vi "minicryo_H-full_202102.vi"() -> ()   [LabVIEW 2013]
uses:
  subVI/B_Globals.vi
  <vilib>/Analysis/NI_AALPro.lvlib
panel:
  out "Numeric":i32
  out "Set Field [T]":dbl
  out "Set Rate [T]":dbl=0.21275819999999998
  out "Exec Time [ms]":u32=526
  out "Stable":bool=TRUE
  out "Act. Rate [T/min]":dbl=-2.1033442988388268e-05
  out "Read Buffer":string="45:85:76 OUTPUT: 0.00000 TESLA AT 0.0 VOLTS \r\n"
  in  "stop":bool
  out "Its":i32=853
  out "Running Sequence":bool
  in  "Set Field":dbl
  in  "Rate":dbl=0.2
  in  "Go To":bool
  out "Field [T]":dbl
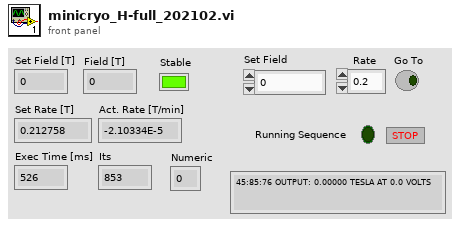
[diagram p1: front panel]
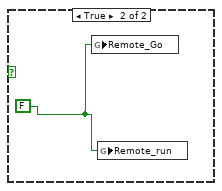
[diagram p2: hidden frame]
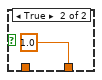
[diagram p3: hidden frame]
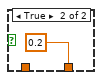
[diagram p4: hidden frame]
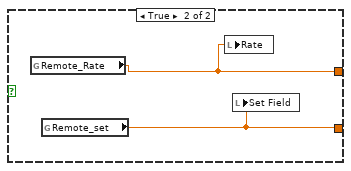
[diagram p5: hidden frame]
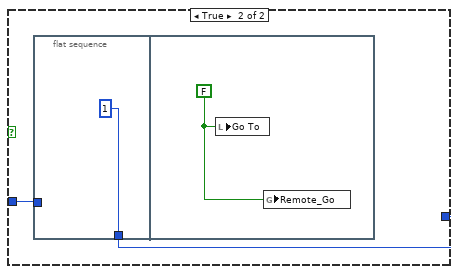
[diagram p6: hidden frame]
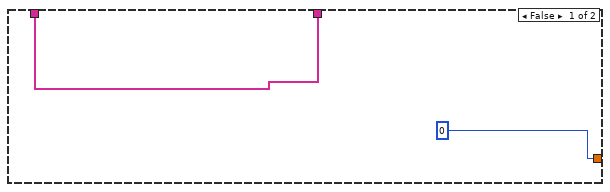
[diagram p7: hidden frame]
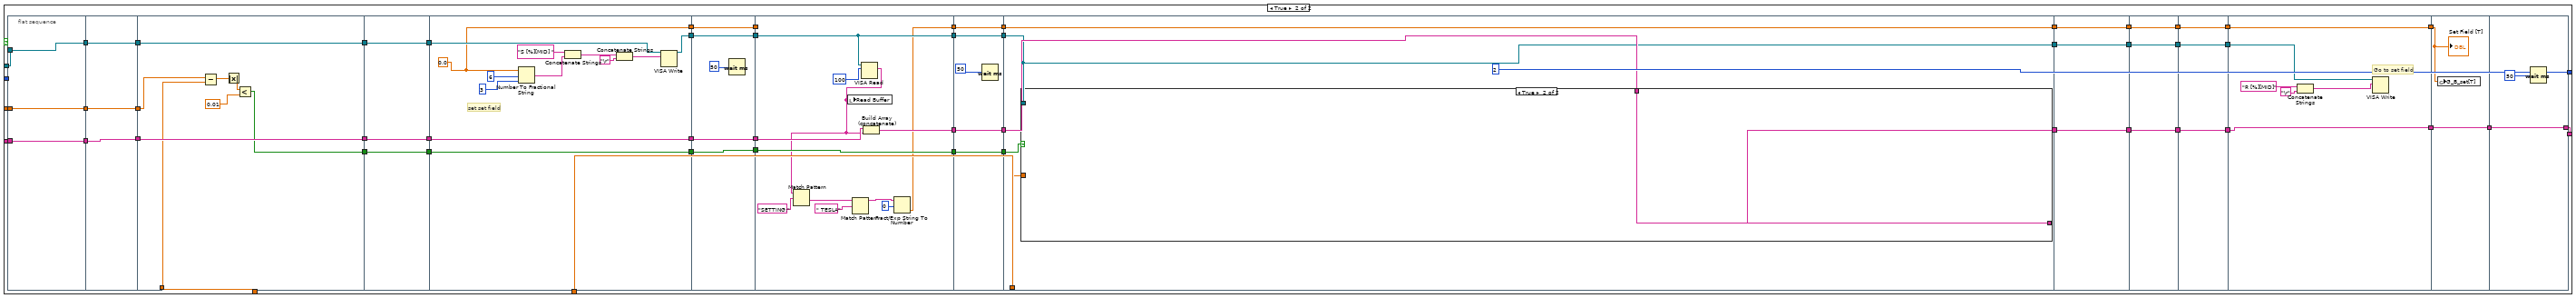
[diagram p10: hidden frame]
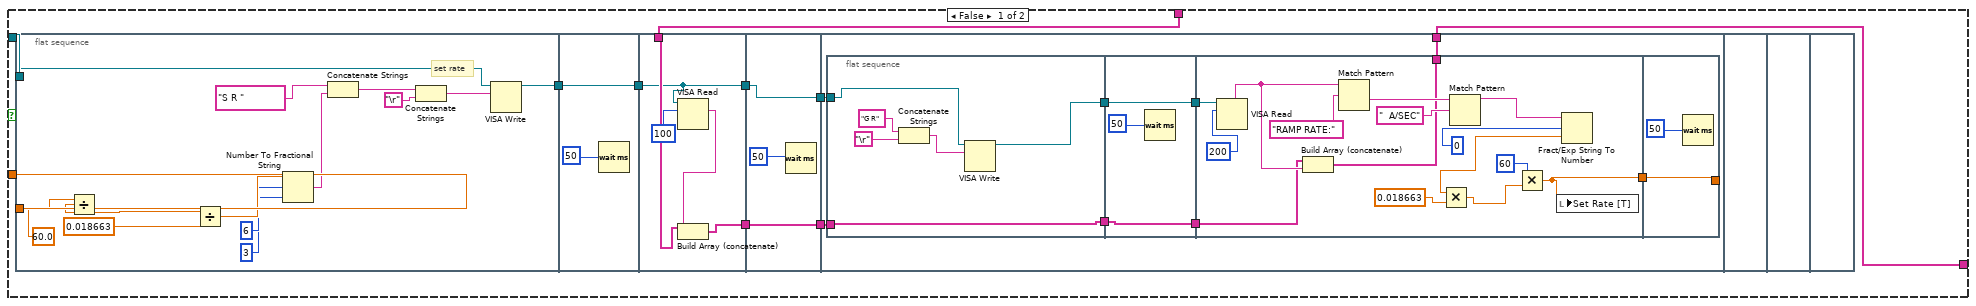
[diagram p11: hidden frame]
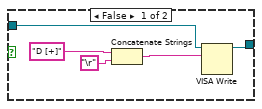
[diagram p14: hidden frame]
diagram:
  n1 = Tick Count (ms)() -> (millisecond timer value=w2:u32)
  n2 = VISA Clear(VISA resource name=refnum<visa-resource-name> "COM7" ("Lakeshore Address")) -> (VISA resource name out=w3:refnum<visa-resource-name>)  [unwired: 1 in, 1 out]
  n3 = while {
    shift-right: [w134] -> _
    shift-left: _ -> [w135]
    shift-right: [w131] -> _
    shift-left: _ -> [w132]
    tunnel: w3 -> [w136]
    shift-right: [w127] -> _
    shift-left: 0 -> [w93]
    shift-right: [w114] -> _
    shift-left: w2 -> [w113]
    shift-right: [w68] -> _
    shift-left: _ -> [w77]
    i -> [w124]
    stop <- FALSE stop-if-true
    n4 = flat-sequence {
      tunnel: w93 -> [w137]
      tunnel: w132 -> [w140]
      tunnel: w135 -> [w142]
      tunnel: w136 -> [w146]
      tunnel: [w146] -> w92
      tunnel: [w143] -> w91
      tunnel: [w139] -> w90
      tunnel: [w137] -> w89
      tunnel: [w138] -> w78
      tunnel: w77 -> [w138]
      tunnel: [w154] -> w118
      tunnel: [w153] -> w117
      tunnel: [w152] -> w116
      tunnel: [w151] -> w115
      tunnel: [w149] -> w114
      tunnel: w113 -> [w148]
      tunnel: w92 -> [w154]
      tunnel: w91 -> [w153]
      tunnel: w90 -> [w152]
      tunnel: w89 -> [w151]
      tunnel: w78 -> [w147]
      tunnel: [w147] -> w74
      tunnel: [w161] -> w88
      tunnel: [w160] -> w86
      tunnel: [w159] -> w84
      tunnel: [w158] -> w82
      tunnel: [w156] -> w80
      tunnel: w118 -> [w161]
      tunnel: w117 -> [w160]
      tunnel: w116 -> [w159]
      tunnel: w115 -> [w158]
      tunnel: [w155] -> w75
      tunnel: w74 -> [w155]
      tunnel: w88 -> [w164]
      tunnel: [w163] -> w87
      tunnel: w86 -> [w169]
      tunnel: [w169] -> w85
      tunnel: w84 -> [w168]
      tunnel: [w168] -> w83
      tunnel: w82 -> [w167]
      tunnel: [w167] -> w81
      tunnel: w80 -> [w166]
      tunnel: [w166] -> w79
      tunnel: [w165] -> w76
      tunnel: w75 -> [w165]
      tunnel: w87 -> [w170]
      tunnel: [w170] -> w123
      tunnel: w85 -> [w176]
      tunnel: [w176] -> w122
      tunnel: w83 -> [w175]
      tunnel: [w175] -> w121
      tunnel: w81 -> [w174]
      tunnel: [w174] -> w120
      tunnel: w79 -> [w173]
      tunnel: [w173] -> w119
      tunnel: w76 -> [w171]
      tunnel: [w171] -> w72
      tunnel: [w186] -> w112
      tunnel: [w185] -> w111
      tunnel: [w183] -> w110
      tunnel: [w184] -> w109
      tunnel: [w179] -> w108
      tunnel: w123 -> [w179]
      tunnel: w122 -> [w186]
      tunnel: w121 -> [w185]
      tunnel: w120 -> [w184]
      tunnel: w119 -> [w183]
      tunnel: [w178] -> w94
      tunnel: [w177] -> w73
      tunnel: w72 -> [w177]
      tunnel: w112 -> [w194]
      tunnel: [w194] -> w25
      tunnel: w111 -> [w193]
      tunnel: [w193] -> w24
      tunnel: w110 -> [w192]
      tunnel: [w192] -> w23
      tunnel: w109 -> [w191]
      tunnel: [w191] -> w22
      tunnel: w108 -> [w190]
      tunnel: [w190] -> w21
      tunnel: [w188] -> w20
      tunnel: w94 -> [w188]
      tunnel: w73 -> [w187]
      tunnel: [w187] -> w19
      tunnel: w25 -> [w201]
      tunnel: [w201] -> w18
      tunnel: w24 -> [w200]
      tunnel: [w200] -> w16
      tunnel: w23 -> [w199]
      tunnel: [w199] -> w14
      tunnel: w22 -> [w198]
      tunnel: [w198] -> w12
      tunnel: w21 -> [w197]
      tunnel: [w197] -> w10
      tunnel: w20 -> [w195]
      tunnel: [w195] -> w8
      tunnel: w19 -> [w196]
      tunnel: [w196] -> w6
      tunnel: w18 -> [w209]
      tunnel: [w209] -> w17
      tunnel: w16 -> [w208]
      tunnel: [w208] -> w15
      tunnel: w14 -> [w207]
      tunnel: [w207] -> w13
      tunnel: w12 -> [w206]
      tunnel: [w206] -> w11
      tunnel: w10 -> [w205]
      tunnel: [w205] -> w9
      tunnel: w8 -> [w204]
      tunnel: [w204] -> w7
      tunnel: w6 -> [w203]
      tunnel: [w203] -> w5
      tunnel: [w214] -> w107
      tunnel: w17 -> [w225]
      tunnel: [w225] -> w106
      tunnel: w15 -> [w224]
      tunnel: [w224] -> w105
      tunnel: w13 -> [w223]
      tunnel: [w223] -> w104
      tunnel: w11 -> [w222]
      tunnel: [w222] -> w103
      tunnel: w9 -> [w221]
      tunnel: [w221] -> w102
      tunnel: [w213] -> w101
      tunnel: w7 -> [w212]
      tunnel: [w211] -> w71
      tunnel: w5 -> [w211]
      tunnel: [w210] -> w26
      tunnel: [w235] -> w49
      tunnel: [w230] -> w48
      tunnel: [w234] -> w47
      tunnel: [w233] -> w46
      tunnel: [w232] -> w45
      tunnel: [w231] -> w44
      tunnel: w107 -> [w230]
      tunnel: w106 -> [w231]
      tunnel: w105 -> [w233]
      tunnel: w104 -> [w232]
      tunnel: w103 -> [w235]
      tunnel: w102 -> [w234]
      tunnel: w101 -> [w229]
      tunnel: w71 -> [w227]
      tunnel: [w228] -> w43
      tunnel: [w226] -> w27
      tunnel: w26 -> [w226]
      tunnel: w49 -> [w244]
      tunnel: [w244] -> w42
      tunnel: w48 -> [w243]
      tunnel: [w243] -> w40
      tunnel: w47 -> [w242]
      tunnel: [w242] -> w38
      tunnel: w46 -> [w241]
      tunnel: [w241] -> w36
      tunnel: w45 -> [w240]
      tunnel: [w240] -> w34
      tunnel: w44 -> [w239]
      tunnel: [w239] -> w32
      tunnel: w43 -> [w238]
      tunnel: [w238] -> w30
      tunnel: [w237] -> w28
      tunnel: w27 -> [w237]
      tunnel: w42 -> [w251]
      tunnel: [w251] -> w41
      tunnel: w40 -> [w250]
      tunnel: [w250] -> w39
      tunnel: w38 -> [w249]
      tunnel: [w249] -> w37
      tunnel: w36 -> [w248]
      tunnel: [w248] -> w35
      tunnel: w34 -> [w247]
      tunnel: [w247] -> w33
      tunnel: w32 -> [w246]
      tunnel: [w246] -> w31
      tunnel: w30 -> [w245]
      tunnel: [w245] -> w29
      tunnel: w28 -> [_]
      tunnel: w41 -> [w259]
      tunnel: [w259] -> w100
      tunnel: w39 -> [w258]
      tunnel: [w258] -> w99
      tunnel: w37 -> [w257]
      tunnel: [w257] -> w98
      tunnel: w35 -> [w256]
      tunnel: [w256] -> w97
      tunnel: w33 -> [w255]
      tunnel: [w255] -> w96
      tunnel: w31 -> [w254]
      tunnel: [w254] -> w95
      tunnel: [w252] -> w70
      tunnel: w29 -> [w252]
      tunnel: [w280] -> w130
      tunnel: [w278] -> w129
      tunnel: [w288] -> w128
      tunnel: w100 -> [w288]
      tunnel: [w283] -> w126
      tunnel: w99 -> [w283]
      tunnel: [w287] -> w125
      tunnel: w98 -> [w287]
      tunnel: w97 -> [w286]
      tunnel: w96 -> [w285]
      tunnel: w95 -> [w284]
      tunnel: w70 -> [w270]
      tunnel: [w270] -> w69
      tunnel: w130 -> [w307]
      tunnel: w129 -> [w306]
      tunnel: w128 -> [w302]
      tunnel: [w307] -> w67
      tunnel: [w306] -> w65
      tunnel: [w301] -> w63
      tunnel: [w300] -> w61
      tunnel: w126 -> [w300]
      tunnel: w125 -> [w299]
      tunnel: [w299] -> w59
      tunnel: [w289] -> w57
      tunnel: [w293] -> w55
      tunnel: [w297] -> w53
      tunnel: w69 -> [w297]
      tunnel: w67 -> [w335]
      tunnel: [w335] -> w66
      tunnel: w65 -> [w334]
      tunnel: [w334] -> w64
      tunnel: w63 -> [w324]
      tunnel: [w324] -> w62
      tunnel: w61 -> [w333]
      tunnel: [w333] -> w60
      tunnel: w59 -> [w330]
      tunnel: [w330] -> w58
      tunnel: w57 -> [w332]
      tunnel: [w332] -> w56
      tunnel: w55 -> [w331]
      tunnel: [w331] -> w54
      tunnel: w53 -> [w329]
      tunnel: [w328] -> w52
      tunnel: [w326] -> w51
      tunnel: [w321] -> w50
      tunnel: [w379] -> w131
      tunnel: [w380] -> w134
      tunnel: w66 -> [w380]
      tunnel: w64 -> [w379]
      tunnel: w62 -> [w373]
      tunnel: [w378] -> w127
      tunnel: w60 -> [w377]
      tunnel: w58 -> [w376]
      tunnel: w56 -> [w375]
      tunnel: w54 -> [w374]
      tunnel: [w372] -> w68
      tunnel: w52 -> [w371]
      tunnel: w51 -> [w370]
      tunnel: w50 -> [w369]
      frame #0 {
        n5 = Array Size(array=w142) -> (size(s)=w145:i32)
        n6 = Subtract(x=w145, y=1000) -> (x-y=w141:i32)
        n7 = Array Subset(array=w142, index=w141) -> (w143:dbl[])  [unwired: 1 in]
        n8 = Array Subset(array=w140, index=w141) -> (w139:dbl[])  [unwired: 1 in]
        "Numeric" <- w137
      }
      frame #1 {
        n9 = Tick Count (ms)() -> (millisecond timer value=w149:u32)
        n10 = Subtract(x=w149, y=w148) -> (x-y=→"Exec Time [ms]":u32)
      }
      frame #2 {
        n11 = case shown="False" "stop" {
          frame False {
          }
          frame True {
            w162 = FALSE
            n12 = global write "B_Globals.vi" "Remote_Go"(w162) -> ()
            n13 = global write "B_Globals.vi" "Remote_run"(w162) -> ()
          }
        }
        n14 = call <vilib>:"High Resolution Relative Seconds.vi"() -> ("relative seconds"=w156:dbl)
      }
      frame #3 {
        n15 = VISA Clear(VISA resource name=w164) -> (VISA resource name out=w163:refnum<visa-resource-name>)  [unwired: 1 in, 1 out]
      }
      frame #4 {
        n16 = Wait (ms)(milliseconds to wait=u32 20 ("Pre Delay")) -> ()  [unwired: 1 out]
      }
      frame #5 {
        n17 = Concatenate Strings("GET OUTPUT " ("Command"), "\r") -> (w181:string)
        n18 = VISA Write(VISA resource name=w179, write buffer=w181) -> (VISA resource name out=w178:refnum<visa-resource-name>)  [unwired: 1 in, 2 out]
      }
      frame #6 {
        n19 = Wait (ms)(milliseconds to wait=u32 50 ("Pre Delay")) -> ()  [unwired: 1 out]
      }
      frame #7 {
      }
      frame #8 {
        n20 = Wait (ms)(milliseconds to wait=u32 50 ("Pre Delay")) -> ()  [unwired: 1 out]
      }
      frame #9 {
        n21 = VISA Read(VISA resource name=w212, byte count=u32 100) -> (VISA resource name out=w210:refnum<visa-resource-name>, read buffer=w213:string)  [unwired: 1 in, 2 out]
        n22 = Match Pattern(string=w213, regular expression="OUTPUT:") -> (after substring=w216:string)  [unwired: 1 in, 3 out]
        n23 = Match Pattern(string=w216, regular expression=" TESLA") -> (before substring=w215:string)  [unwired: 1 in, 3 out]
        n24 = Fract/Exp String To Number(string=w215, offset=0) -> (number=w214:dbl)  [unwired: 2 in, 1 out]
      }
      frame #10 {
        n25 = global write "B_Globals.vi" "B [T]"(w230) -> ()
        n26 = Build Array (concatenate)(w227, w229) -> (w228:string[])
        "Field [T]" <- w230
        "Read Buffer" <- w229
      }
      frame #11 {
        n27 = Wait (ms)(milliseconds to wait=u32 0 ("Pre Delay")) -> ()  [unwired: 1 out]
      }
      frame #12 {
      }
      frame #13 {
        n28 = Wait (ms)(milliseconds to wait=u32 100 ("Pre Delay")) -> ()  [unwired: 1 out]
      }
      frame #14 {
        n29 = Build Array (concatenate)(w284, w283) -> (w280:dbl[])
        n30 = Build Array (concatenate)(w286, w285) -> (w278:dbl[])
        n31 = Array Size(array=w280) -> (size(s)=w281:i32)
        n32 = Subtract(x=w281, y=50) -> (x-y=w279:i32)
        n33 = Array Subset(array=w278, index=w279) -> (w276:dbl[])  [unwired: 1 in]
        n34 = Array Subset(array=w280, index=w279) -> (w277:dbl[])  [unwired: 1 in]
        n35 = call <vilib>:"Linear Fit.vi"("Y"=w277, "X"=w276) -> ("slope"=w272:dbl)  [unwired: 9 in, 4 out]
        n36 = local read "Set Field [T]"() -> (w263:dbl)
        n37 = local read "Field [T]"() -> (w262:dbl)
        n38 = Multiply(x=w272, y=60) -> (x*y=w271:dbl)
        "Act. Rate [T/min]" <- w271
        n39 = Absolute Value(x=w263) -> (abs(x)=w260:dbl)
        n40 = Absolute Value(x=w262) -> (abs(x)=w261:dbl)
        n41 = Subtract(x=w260, y=w261) -> (x-y=w269:dbl)
        n42 = Absolute Value(x=w271) -> (abs(x)=w273:dbl)
        n43 = Less?(x=w273, y=0.01) -> (x < y?=w265:bool)
        n44 = Absolute Value(x=w269) -> (abs(x)=w268:dbl)
        n45 = Less?(x=w268, y=0.02) -> (x < y?=w264:bool)
        n46 = And(x=w265, y=w264) -> (x .and. y?=w266:bool)
        "Stable" <- w266
        n47 = global write "B_Globals.vi" "Rem_stable_B"(w266) -> ()
      }
      frame #15 {
        n48 = global read "B_Globals.vi" "Remote_Go"() -> (w305:bool)
        n49 = global read "B_Globals.vi" "Remote_run"() -> (w298:bool)
        "Running Sequence" <- w298
        n50 = Or(x=w305, y="Go To") -> (x .or. y?=w303:bool)
        n51 = case shown="False" w303 {
          tunnel: w302 -> [w316 w318]
          tunnel: [w316 w317] -> w301
          frame False {
          }
          frame True {
            n52 = flat-sequence {
              tunnel: w318 -> [_]
              tunnel: [1] -> w317
              frame #0 {
              }
              frame #1 {
                w320 = FALSE
                n53 = local write "Go To"(w320) -> ()
                n54 = global write "B_Globals.vi" "Remote_Go"(w320) -> ()
              }
            }
          }
        }
        n55 = case shown="False" w298 {
          tunnel: ["Set Field" w314] -> w290
          tunnel: ["Rate" w315] -> w294
          frame False {
          }
          frame True {
            n56 = global read "B_Globals.vi" "Remote_Rate"() -> (w315:dbl)
            n57 = global read "B_Globals.vi" "Remote_set"() -> (w314:dbl)
            n58 = local write "Rate"(w315) -> ()
            n59 = local write "Set Field"(w314) -> ()
          }
        }
        n60 = Greater?(x=w294, y=0.2) -> (0:w295:bool)
        n61 = Greater?(x=w290, y=1.0) -> (0:w291:bool)
        n62 = case shown="False" w291 {
          tunnel: [w308 1.0] -> w289
          tunnel: w290 -> [w308 _]
          frame False {
          }
          frame True {
          }
        }
        n63 = case shown="False" w295 {
          tunnel: [w310 0.2] -> w293
          tunnel: w294 -> [w310 _]
          frame False {
          }
          frame True {
          }
        }
      }
      frame #16 {
        n64 = Not Equal?(x=0, y=w324) -> (x != y?=w321:bool)
        n65 = Not Equal?(x=w324, y=2) -> (x != y?=w323:bool)
        n66 = And(x=w323, y=w321) -> (x .and. y?=w322:bool)
        n67 = case shown="True" w322 {
          tunnel: w330 -> [_ w342]
          tunnel: w329 -> [w337 w341]
          tunnel: [w337 w340] -> w328
          tunnel: [0 w338] -> w326
          frame False {
          }
          frame True {
            n68 = flat-sequence {
              tunnel: w342 -> [w346]
              tunnel: [w345] -> w344
              tunnel: w344 -> [w350]
              tunnel: [w350] -> w343
              tunnel: w343 -> [w363]
              tunnel: w341 -> [w360]
              tunnel: [w359] -> w340
              tunnel: [w352] -> w339
              tunnel: [w367] -> w338
              tunnel: w339 -> [w367]
              frame #0 {
                n69 = Concatenate Strings("G R" ("Command"), "\r") -> (w348:string)
                n70 = VISA Write(VISA resource name=w346, write buffer=w348) -> (VISA resource name out=w345:refnum<visa-resource-name>)  [unwired: 1 in, 2 out]
              }
              frame #1 {
                n71 = Wait (ms)(milliseconds to wait=100) -> ()  [unwired: 1 out]
              }
              frame #2 {
                (unwired) 0.018663 ("y")
                n72 = VISA Read(VISA resource name=w363, byte count=u32 200) -> (read buffer=w361:string)  [unwired: 1 in, 3 out]
                n73 = Build Array (concatenate)(w360, w361) -> (w359:string[])
                n74 = Match Pattern(string=w361, regular expression="RAMP RATE:") -> (after substring=w364:string)  [unwired: 1 in, 3 out]
                n75 = Match Pattern(string=w364, regular expression="  A/SEC") -> (before substring=w357:string)  [unwired: 1 in, 3 out]
                n76 = Fract/Exp String To Number(string=w357, offset=0) -> (number=w355:dbl)  [unwired: 2 in, 1 out]
                n77 = Multiply(x=w355, y=0.018663) -> (x*y=w353:dbl)
                n78 = Multiply(x=60, y=w353) -> (x*y=w352:dbl)
                "Set Rate [T]" <- w352
              }
              frame #3 {
                n79 = Wait (ms)(milliseconds to wait=100) -> ()  [unwired: 1 out]
              }
            }
          }
        }
      }
      frame #17 {
        # "Bnow"
        # "Barray"
        n80 = case shown="3" w373 {
          tunnel: w377 -> [_ w399 w606 _ _]
          tunnel: w373 -> [w383 w392 w603 _ _]
          tunnel: [w383 w391 w602 4 w715] -> w378
          tunnel: w374 -> [_ w384 _ _ w717]
          tunnel: w376 -> [_ w388 _ w625 w713]
          tunnel: w375 -> [_ w389 _ _ w714]
          tunnel: w371 -> [w381 w387 w601 w621 w698]
          tunnel: [w381 w386 w601 w626 w692] -> w372
          tunnel: w370 -> [_ w385 _ _ _]
          tunnel: w369 -> [_ _ _ _ _]
          frame 0, Default {
            n81 = Wait (ms)(milliseconds to wait=0) -> ()  [unwired: 1 out]
          }
          frame 1 {
            # "If True need to reverse polarity"
            n82 = Less Than 0?(x=w389) -> (x < 0?=w390:bool)
            n83 = Number To Fractional String(number=w399) -> (F-format string=w402:string)  [unwired: 3 in]
            n84 = String Subset(string=w402, length (rest)=1 ("length (rest)")) -> (substring=w401:string)  [unwired: 1 in]
            n85 = Equal?(x=w401, y="-") -> (x = y?=w394:bool)
            n86 = Not Or(1:w390, 2:w394) -> (0:w398:bool)
            n87 = Not Or(1:w398, 2:w394) -> (0:w397:bool)
            n88 = Not Or(1:w390, 2:w398) -> (0:w396:bool)
            n89 = Not Or(1:w396, 2:w397) -> (0:w395:bool)
            n90 = Not(x=w395) -> (.not. x?=w393:bool)
            n91 = case shown="False" w393 {
              tunnel: w392 -> [_ _]
              tunnel: [4 2] -> w391
              tunnel: w384 -> [_ w453]
              tunnel: w388 -> [_ w451]
              tunnel: w387 -> [w404 w442]
              tunnel: [w404 w433] -> w386
              tunnel: w385 -> [_ w414]
              tunnel: w384 -> [_ w412]
              frame False {
              }
              frame True {
                n92 = flat-sequence {
                  tunnel: w451 -> [w457]
                  tunnel: [w457] -> w450
                  tunnel: [w458] -> w443
                  tunnel: w442 -> [w458]
                  tunnel: [w456] -> w415
                  tunnel: w414 -> [w456]
                  tunnel: [w461] -> w421
                  tunnel: w450 -> [w461]
                  tunnel: w443 -> [w460]
                  tunnel: [w460] -> w420
                  tunnel: w415 -> [w459]
                  tunnel: [w459] -> w413
                  tunnel: w421 -> [w469]
                  tunnel: [w469] -> w419
                  tunnel: w420 -> [w468]
                  tunnel: [w468] -> w417
                  tunnel: w413 -> [w467]
                  tunnel: w412 -> [w466]
                  tunnel: [w462] -> w411
                  tunnel: w419 -> [w472]
                  tunnel: [w472] -> w418
                  tunnel: w417 -> [w471]
                  tunnel: [w471] -> w416
                  tunnel: w411 -> [w470]
                  tunnel: [w470] -> w410
                  tunnel: [w477] -> w454
                  tunnel: w418 -> [w476]
                  tunnel: [w475] -> w440
                  tunnel: w416 -> [w475]
                  tunnel: [w474] -> w422
                  tunnel: w410 -> [w473]
                  tunnel: [w473] -> w409
                  tunnel: [w488] -> w449
                  tunnel: w454 -> [w488]
                  tunnel: [w487] -> w441
                  tunnel: w440 -> [w487]
                  tunnel: [w486] -> w423
                  tunnel: w422 -> [w486]
                  tunnel: w409 -> [w485]
                  tunnel: [w485] -> w408
                  tunnel: w449 -> [w500]
                  tunnel: [w500] -> w448
                  tunnel: w441 -> [w499]
                  tunnel: [w498] -> w438
                  tunnel: [w490] -> w424
                  tunnel: w423 -> [_]
                  tunnel: w408 -> [w497]
                  tunnel: [w497] -> w407
                  tunnel: w448 -> [w506]
                  tunnel: [w506] -> w447
                  tunnel: [w504] -> w439
                  tunnel: w438 -> [w504]
                  tunnel: [w503] -> w425
                  tunnel: w424 -> [w503]
                  tunnel: w407 -> [w502]
                  tunnel: [w502] -> w406
                  tunnel: w447 -> [w507]
                  tunnel: w453 -> [w512]
                  tunnel: [w507] -> w452
                  tunnel: w439 -> [w508]
                  tunnel: [w509] -> w436
                  tunnel: [w511] -> w426
                  tunnel: w425 -> [w511]
                  tunnel: w406 -> [w510]
                  tunnel: [w584] -> w446
                  tunnel: w452 -> [w584]
                  tunnel: [w583] -> w437
                  tunnel: w436 -> [w583]
                  tunnel: [w582] -> w427
                  tunnel: w426 -> [w582]
                  tunnel: w446 -> [w587]
                  tunnel: [w587] -> w445
                  tunnel: w437 -> [w585]
                  tunnel: [w585] -> w434
                  tunnel: [w586] -> w428
                  tunnel: w427 -> [w586]
                  tunnel: w445 -> [w590]
                  tunnel: [w590] -> w444
                  tunnel: [w589] -> w435
                  tunnel: w434 -> [w589]
                  tunnel: [w588] -> w429
                  tunnel: w428 -> [w588]
                  tunnel: w444 -> [w593]
                  tunnel: w435 -> [w592]
                  tunnel: [w592] -> w432
                  tunnel: [w591] -> w430
                  tunnel: w429 -> [w591]
                  tunnel: w432 -> [w598]
                  tunnel: [w598] -> w431
                  tunnel: w430 -> [w597]
                  tunnel: [w599] -> w433
                  tunnel: w431 -> [w599]
                  frame #0 {
                  }
                  frame #1 {
                  }
                  frame #2 {
                    n93 = Subtract(x=w467, y=w466) -> (x-y=w465:dbl)
                    n94 = Absolute Value(x=w465) -> (abs(x)=w464:dbl)
                    n95 = Less?(x=w464, y=0.01) -> (x < y?=w462:bool)
                  }
                  frame #3 {
                  }
                  frame #4 {
                    w474 = 0.0
                    # "set set field"
                    n96 = Number To Fractional String(number=w474, width (-)=i16 6, precision (6)=i16 3) -> (F-format string=w481:string)  [unwired: 1 in]
                    n97 = Concatenate Strings("S [%][MID] " ("string"), w481) -> (w478:string)
                    n98 = Concatenate Strings(w478, "\r") -> (w480:string)
                    n99 = VISA Write(VISA resource name=w476, write buffer=w480) -> (VISA resource name out=w477:refnum<visa-resource-name>)  [unwired: 1 in, 2 out]
                  }
                  frame #5 {
                    n100 = Wait (ms)(milliseconds to wait=50) -> ()  [unwired: 1 out]
                  }
                  frame #6 {
                    n101 = VISA Read(VISA resource name=w500, byte count=100) -> (read buffer=w491:string)  [unwired: 1 in, 3 out]
                    n102 = Match Pattern(string=w491, regular expression="SETTING:") -> (after substring=w495:string)  [unwired: 1 in, 3 out]
                    n103 = local write "Read Buffer"(w491) -> ()
                    n104 = Match Pattern(string=w495, regular expression=" TESLA") -> (before substring=w496:string)  [unwired: 1 in, 3 out]
                    n105 = Build Array (concatenate)(w499, w491) -> (w498:string[])
                    n106 = Fract/Exp String To Number(string=w496, offset=0) -> (number=w490:dbl)  [unwired: 2 in, 1 out]
                  }
                  frame #7 {
                    n107 = Wait (ms)(milliseconds to wait=50) -> ()  [unwired: 1 out]
                  }
                  frame #8 {
                    n108 = case shown="True" w510 {
                      tunnel: w507 -> [w522 _]
                      tunnel: w512 -> [w521 _]
                      tunnel: w508 -> [w517 w581]
                      tunnel: [w514 w581] -> w509
                      frame False {
                        n109 = flat-sequence {
                          tunnel: w522 -> [w525]
                          tunnel: w521 -> [w524]
                          tunnel: [w523] -> w520
                          tunnel: w520 -> [w538]
                          tunnel: [w538] -> w519
                          tunnel: w519 -> [w540]
                          tunnel: [w540] -> w518
                          tunnel: w517 -> [w541]
                          tunnel: [w539] -> w515
                          tunnel: w518 -> [w544]
                          tunnel: [w545] -> w516
                          tunnel: w515 -> [w545]
                          tunnel: [w544] -> w513
                          tunnel: w516 -> [w551]
                          tunnel: [w548] -> w514
                          tunnel: w513 -> [w547]
                          frame #0 {
                            # "set rate"
                            n110 = Divide(x=w524, y=60.0) -> (x/y=w530:dbl)
                            n111 = Divide(x=w530, y=0.018663) -> (x/y=w528:dbl)
                            n112 = Number To Fractional String(number=w528, width (-)=i16 6, precision (6)=i16 3) -> (F-format string=w533:string)  [unwired: 1 in]
                            n113 = Concatenate Strings("S R " ("string"), w533) -> (w532:string)
                            n114 = Concatenate Strings(w532, "\r") -> (w536:string)
                            n115 = VISA Write(VISA resource name=w525, write buffer=w536) -> (VISA resource name out=w523:refnum<visa-resource-name>)  [unwired: 1 in, 2 out]
                          }
                          frame #1 {
                            n116 = Wait (ms)(milliseconds to wait=50) -> ()  [unwired: 1 out]
                          }
                          frame #2 {
                            n117 = VISA Read(VISA resource name=w540, byte count=100) -> (read buffer=w542:string)  [unwired: 1 in, 3 out]
                            n118 = Build Array (concatenate)(w541, w542) -> (w539:string[])
                          }
                          frame #3 {
                            n119 = Wait (ms)(milliseconds to wait=50) -> ()  [unwired: 1 out]
                          }
                          frame #4 {
                            n120 = flat-sequence {
                              tunnel: [w557] -> w554
                              tunnel: w551 -> [w556]
                              tunnel: [w556] -> w549
                              tunnel: w547 -> [w555]
                              tunnel: w554 -> [w562]
                              tunnel: [w562] -> w553
                              tunnel: [w561] -> w550
                              tunnel: w549 -> [w561]
                              tunnel: w553 -> [w575]
                              tunnel: [w572] -> w548
                              tunnel: [w565] -> w552
                              tunnel: w550 -> [w564]
                              tunnel: [w579] -> _
                              tunnel: w552 -> [w579]
                              frame #0 {
                                n121 = Concatenate Strings("G R" ("Command"), "\r") -> (w559:string)
                                n122 = VISA Write(VISA resource name=w555, write buffer=w559) -> (VISA resource name out=w557:refnum<visa-resource-name>)  [unwired: 1 in, 2 out]
                              }
                              frame #1 {
                                n123 = Wait (ms)(milliseconds to wait=50) -> ()  [unwired: 1 out]
                              }
                              frame #2 {
                                n124 = VISA Read(VISA resource name=w575, byte count=u32 200) -> (read buffer=w573:string)  [unwired: 1 in, 3 out]
                                n125 = Build Array (concatenate)(w564, w573) -> (w572:string[])
                                n126 = Match Pattern(string=w573, regular expression="RAMP RATE:") -> (after substring=w576:string)  [unwired: 1 in, 3 out]
                                n127 = Match Pattern(string=w576, regular expression="  A/SEC") -> (before substring=w570:string)  [unwired: 1 in, 3 out]
                                n128 = Fract/Exp String To Number(string=w570, offset=0) -> (number=w568:dbl)  [unwired: 2 in, 1 out]
                                n129 = Multiply(x=w568, y=0.018663) -> (x*y=w566:dbl)
                                n130 = Multiply(x=60, y=w566) -> (x*y=w565:dbl)
                                n131 = local write "Set Rate [T]"(w565) -> ()
                              }
                              frame #3 {
                                n132 = Wait (ms)(milliseconds to wait=50) -> ()  [unwired: 1 out]
                              }
                            }
                          }
                          frame #5 {
                          }
                          frame #6 {
                          }
                          frame #7 {
                          }
                        }
                      }
                      frame True {
                      }
                    }
                  }
                  frame #9 {
                  }
                  frame #10 {
                  }
                  frame #11 {
                  }
                  frame #12 {
                    # "Go to set field"
                    n133 = Concatenate Strings("R [%][MID]" ("data"), "\r") -> (w596:string)
                    n134 = VISA Write(VISA resource name=w593, write buffer=w596) -> ()  [unwired: 1 in, 3 out]
                  }
                  frame #13 {
                    n135 = global write "B_Globals.vi" "G_B_set[T]"(w597) -> ()
                    "Set Field [T]" <- w597
                  }
                  frame #14 {
                    n136 = Wait (ms)(milliseconds to wait=50) -> ()  [unwired: 1 out]
                  }
                }
              }
            }
          }
          frame 2 {
            # "Awaiting 0 Field"
            n137 = Subtract(x=w606, y=0) -> (x-y=w608:dbl)
            n138 = Absolute Value(x=w608) -> (abs(x)=w605:dbl)
            n139 = Less?(x=w605, y=0.001) -> (x < y?=w604:bool)
            n140 = case shown="True" w604 {
              tunnel: w603 -> [w610 _]
              tunnel: [w610 3] -> w602
              frame False {
              }
              frame True {
                # "Close to 0"
                n141 = Wait (ms)(milliseconds to wait=1000) -> ()  [unwired: 1 out]
              }
            }
          }
          frame 3 {
            n142 = flat-sequence {
              tunnel: w625 -> [w630]
              tunnel: [w630] -> w624
              tunnel: w624 -> [w636]
              tunnel: [w635] -> w623
              tunnel: w623 -> [w638]
              tunnel: [w638] -> w622
              tunnel: w622 -> [w648]
              tunnel: [w648] -> w618
              tunnel: w621 -> [w646]
              tunnel: [w645] -> w616
              tunnel: [w641] -> w613
              tunnel: w618 -> [w652]
              tunnel: [w652] -> w617
              tunnel: w616 -> [w651]
              tunnel: [w651] -> w615
              tunnel: [w649] -> w614
              tunnel: w613 -> [w649]
              tunnel: [w657] -> w628
              tunnel: w617 -> [w658]
              tunnel: w615 -> [w656]
              tunnel: [w656] -> w620
              tunnel: w614 -> [w654]
              tunnel: w628 -> [w671]
              tunnel: [w671] -> w627
              tunnel: w620 -> [w669]
              tunnel: [w669] -> w619
              tunnel: w627 -> [w676]
              tunnel: [w674] -> w626
              tunnel: w619 -> [w672]
              frame #0 {
                n143 = Wait (ms)(milliseconds to wait=500) -> ()  [unwired: 1 out]
              }
              frame #1 {
                n144 = Concatenate Strings("GET S " ("data"), "\r") -> (w632:string)
                n145 = VISA Write(VISA resource name=w636, write buffer=w632) -> (VISA resource name out=w635:refnum<visa-resource-name>)  [unwired: 1 in, 2 out]
              }
              frame #2 {
                n146 = Wait (ms)(milliseconds to wait=50) -> ()  [unwired: 1 out]
              }
              frame #3 {
                n147 = VISA Read(VISA resource name=w648, byte count=100) -> (read buffer=w644:string)  [unwired: 1 in, 3 out]
                n148 = local write "Read Buffer"(w644) -> ()
                n149 = Build Array (concatenate)(w646, w644) -> (w645:string[])
                n150 = Match Pattern(string=w644, regular expression="CURRENT DIRECTION: ") -> (after substring=w642:string)  [unwired: 1 in, 3 out]
                n151 = Search and Replace String(input string=w642, search string="\r\n", replace string="") -> (result string=w641:string)  [unwired: 5 in, 3 out]
              }
              frame #4 {
                n152 = Wait (ms)(milliseconds to wait=50) -> ()  [unwired: 1 out]
              }
              frame #5 {
                (unwired) TRUE
                # "Switch polarity"
                n153 = Equal?(x=w654, y="POSITIVE") -> (x = y?=w653:bool)
                n154 = case shown="True" w653 {
                  tunnel: w658 -> [w659 w665]
                  tunnel: [w660 w664] -> w657
                  frame False {
                    n155 = Concatenate Strings("D [+]" ("data"), "\r") -> (w663:string)
                    n156 = VISA Write(VISA resource name=w659, write buffer=w663) -> (VISA resource name out=w660:refnum<visa-resource-name>)  [unwired: 1 in, 2 out]
                  }
                  frame True {
                    n157 = Concatenate Strings("D [-]" ("data"), "\r") -> (w668:string)
                    n158 = VISA Write(VISA resource name=w665, write buffer=w668) -> (VISA resource name out=w664:refnum<visa-resource-name>)  [unwired: 1 in, 2 out]
                  }
                }
              }
              frame #6 {
                n159 = Wait (ms)(milliseconds to wait=50) -> ()  [unwired: 1 out]
              }
              frame #7 {
                n160 = VISA Read(VISA resource name=w676, byte count=100) -> (read buffer=w673:string)  [unwired: 1 in, 3 out]
                n161 = Build Array (concatenate)(w672, w673) -> (w674:string[])
                n162 = local write "Read Buffer"(w673) -> ()
              }
              frame #8 {
                n163 = Wait (ms)(milliseconds to wait=500) -> ()  [unwired: 1 out]
              }
            }
          }
          frame 4 {
            n164 = flat-sequence {
              tunnel: w713 -> [w720]
              tunnel: [w720] -> w711
              tunnel: [w719] -> w700
              tunnel: w698 -> [w719]
              tunnel: [w722] -> w712
              tunnel: w711 -> [w722]
              tunnel: w700 -> [w721]
              tunnel: [w721] -> w699
              tunnel: [w726] -> w718
              tunnel: w714 -> [w724]
              tunnel: w712 -> [w727]
              tunnel: [w725] -> w702
              tunnel: w699 -> [w725]
              tunnel: [w724] -> w686
              tunnel: [w737] -> w710
              tunnel: w718 -> [w737]
              tunnel: w702 -> [w736]
              tunnel: [w736] -> w701
              tunnel: [w735] -> w687
              tunnel: w686 -> [w735]
              tunnel: w710 -> [w749]
              tunnel: [w749] -> w709
              tunnel: [w747] -> w704
              tunnel: w701 -> [w746]
              tunnel: w687 -> [_]
              tunnel: [w739] -> w678
              tunnel: [w754] -> w682
              tunnel: [w753] -> w681
              tunnel: [w752] -> w680
              tunnel: [w751] -> w679
              tunnel: w717 -> [w751]
              tunnel: w704 -> [w753]
              tunnel: w709 -> [w754]
              tunnel: w678 -> [w752]
              tunnel: w682 -> [w763]
              tunnel: [w763] -> w685
              tunnel: w681 -> [w762]
              tunnel: [w761] -> w684
              tunnel: w680 -> [w764]
              tunnel: [w764] -> w683
              tunnel: w679 -> [w756]
              tunnel: w685 -> [w834]
              tunnel: [w834] -> w706
              tunnel: [w833] -> w703
              tunnel: w684 -> [w833]
              tunnel: [w832] -> w688
              tunnel: w683 -> [w832]
              tunnel: w706 -> [w837]
              tunnel: [w837] -> w705
              tunnel: w703 -> [w836]
              tunnel: [w836] -> w693
              tunnel: [w835] -> w689
              tunnel: w688 -> [w835]
              tunnel: [w840] -> w716
              tunnel: w705 -> [w840]
              tunnel: [w839] -> w694
              tunnel: w693 -> [w839]
              tunnel: [w838] -> w690
              tunnel: w689 -> [w838]
              tunnel: w716 -> [w845]
              tunnel: [0] -> w715
              tunnel: [w843] -> w707
              tunnel: [w842] -> w695
              tunnel: w694 -> [w842]
              tunnel: [w841] -> w691
              tunnel: w690 -> [w841]
              tunnel: [w851] -> w708
              tunnel: w707 -> [w851]
              tunnel: [w850] -> w696
              tunnel: w695 -> [w850]
              tunnel: w691 -> [w849]
              tunnel: w708 -> [_]
              tunnel: [w853] -> w697
              tunnel: w696 -> [w853]
              tunnel: [w854] -> w692
              tunnel: w697 -> [w854]
              frame #0 {
              }
              frame #1 {
                n165 = Wait (ms)(milliseconds to wait=50) -> ()  [unwired: 1 out]
              }
              frame #2 {
                # "set set field"
                n166 = Number To Fractional String(number=w724, width (-)=i16 6, precision (6)=i16 3) -> (F-format string=w731:string)  [unwired: 1 in]
                n167 = Concatenate Strings("S [%][MID] " ("string"), w731) -> (w728:string)
                n168 = Concatenate Strings(w728, "\r") -> (w730:string)
                n169 = VISA Write(VISA resource name=w727, write buffer=w730) -> (VISA resource name out=w726:refnum<visa-resource-name>)  [unwired: 1 in, 2 out]
              }
              frame #3 {
                n170 = Wait (ms)(milliseconds to wait=50) -> ()  [unwired: 1 out]
              }
              frame #4 {
                n171 = VISA Read(VISA resource name=w749, byte count=100) -> (read buffer=w740:string)  [unwired: 1 in, 3 out]
                n172 = Build Array (concatenate)(w746, w740) -> (w747:string[])
                n173 = local write "Read Buffer"(w740) -> ()
                n174 = Match Pattern(string=w740, regular expression="SETTING:") -> (after substring=w744:string)  [unwired: 1 in, 3 out]
                n175 = Match Pattern(string=w744, regular expression=" TESLA") -> (before substring=w745:string)  [unwired: 1 in, 3 out]
                n176 = Fract/Exp String To Number(string=w745, offset=0) -> (number=w739:dbl)  [unwired: 2 in, 1 out]
              }
              frame #5 {
                n177 = Wait (ms)(milliseconds to wait=50) -> ()  [unwired: 1 out]
              }
              frame #6 {
                n178 = local read "Set Rate [T]"() -> (w757:dbl)
                n179 = Subtract(x=w757, y=w756) -> (x-y=w760:dbl)
                n180 = Absolute Value(x=w760) -> (abs(x)=w759:dbl)
                n181 = Less?(x=w759, y=0.01) -> (x < y?=w755:bool)
                n182 = case shown="False" w755 {
                  tunnel: w763 -> [w774 _]
                  tunnel: w756 -> [w773 _]
                  tunnel: [w767 w831] -> w761
                  tunnel: w762 -> [w765 w831]
                  frame False {
                    n183 = flat-sequence {
                      tunnel: w774 -> [w777]
                      tunnel: w773 -> [w776]
                      tunnel: [w775] -> w772
                      tunnel: w772 -> [w790]
                      tunnel: [w790] -> w771
                      tunnel: w771 -> [w793]
                      tunnel: [w793] -> w770
                      tunnel: [w792] -> w768
                      tunnel: w765 -> [w791]
                      tunnel: w770 -> [w796]
                      tunnel: [w797] -> w769
                      tunnel: w768 -> [w797]
                      tunnel: [w796] -> w766
                      tunnel: w769 -> [w803]
                      tunnel: [w800] -> w767
                      tunnel: w766 -> [w799]
                      frame #0 {
                        # "set rate"
                        n184 = Divide(x=w776, y=60.0) -> (x/y=w782:dbl)
                        n185 = Divide(x=w782, y=0.018663) -> (x/y=w780:dbl)
                        n186 = Number To Fractional String(number=w780, width (-)=i16 6, precision (6)=i16 3) -> (F-format string=w785:string)  [unwired: 1 in]
                        n187 = Concatenate Strings("S R " ("string"), w785) -> (w784:string)
                        n188 = Concatenate Strings(w784, "\r") -> (w788:string)
                        n189 = VISA Write(VISA resource name=w777, write buffer=w788) -> (VISA resource name out=w775:refnum<visa-resource-name>)  [unwired: 1 in, 2 out]
                      }
                      frame #1 {
                        n190 = Wait (ms)(milliseconds to wait=50) -> ()  [unwired: 1 out]
                      }
                      frame #2 {
                        n191 = VISA Read(VISA resource name=w793, byte count=100) -> (read buffer=w794:string)  [unwired: 1 in, 3 out]
                        n192 = Build Array (concatenate)(w791, w794) -> (w792:string[])
                      }
                      frame #3 {
                        n193 = Wait (ms)(milliseconds to wait=50) -> ()  [unwired: 1 out]
                      }
                      frame #4 {
                        n194 = flat-sequence {
                          tunnel: [w808] -> w805
                          tunnel: w803 -> [w807]
                          tunnel: [w807] -> w801
                          tunnel: w799 -> [w806]
                          tunnel: w805 -> [w813]
                          tunnel: [w813] -> w804
                          tunnel: [w812] -> w802
                          tunnel: w801 -> [w812]
                          tunnel: w804 -> [w826]
                          tunnel: [w823] -> w800
                          tunnel: w802 -> [w816]
                          frame #0 {
                            n195 = Concatenate Strings("G R" ("Command"), "\r") -> (w810:string)
                            n196 = VISA Write(VISA resource name=w806, write buffer=w810) -> (VISA resource name out=w808:refnum<visa-resource-name>)  [unwired: 1 in, 2 out]
                          }
                          frame #1 {
                            n197 = Wait (ms)(milliseconds to wait=20) -> ()  [unwired: 1 out]
                          }
                          frame #2 {
                            n198 = VISA Read(VISA resource name=w826, byte count=u32 200) -> (read buffer=w824:string)  [unwired: 1 in, 3 out]
                            n199 = Build Array (concatenate)(w816, w824) -> (w823:string[])
                            n200 = Match Pattern(string=w824, regular expression="RAMP RATE:") -> (after substring=w827:string)  [unwired: 1 in, 3 out]
                            n201 = Match Pattern(string=w827, regular expression="  A/SEC") -> (before substring=w821:string)  [unwired: 1 in, 3 out]
                            n202 = Fract/Exp String To Number(string=w821, offset=0) -> (number=w819:dbl)  [unwired: 2 in, 1 out]
                            n203 = Multiply(x=w819, y=0.018663) -> (x*y=w817:dbl)
                            n204 = Multiply(x=60, y=w817) -> (x*y=w815:dbl)
                            n205 = local write "Set Rate [T]"(w815) -> ()
                          }
                          frame #3 {
                            n206 = Wait (ms)(milliseconds to wait=50) -> ()  [unwired: 1 out]
                          }
                        }
                      }
                      frame #5 {
                      }
                      frame #6 {
                      }
                      frame #7 {
                      }
                    }
                  }
                  frame True {
                  }
                }
              }
              frame #7 {
              }
              frame #8 {
              }
              frame #9 {
              }
              frame #10 {
                # "Go to set field"
                n207 = Concatenate Strings("R [%][MID]" ("data"), "\r") -> (w848:string)
                n208 = VISA Write(VISA resource name=w845, write buffer=w848) -> (VISA resource name out=w843:refnum<visa-resource-name>)  [unwired: 1 in, 2 out]
              }
              frame #11 {
                n209 = local write "Set Field [T]"(w849) -> ()
                n210 = global write "B_Globals.vi" "G_B_set[T]"(w849) -> ()
              }
              frame #12 {
                n211 = Wait (ms)(milliseconds to wait=50) -> ()  [unwired: 1 out]
              }
              frame #13 {
              }
            }
          }
        }
      }
    }
    "Its" <- w124
  }
